vi "Launch Test.vi"(5 "timeout ms (-1)":i32=-1, 6 "Station":T1(ring), 8 "error in (no error)":errorcluster, 10 "SerialNumber":string[](array[string]), 11 "Sequence":string) -> (0 "error out":errorcluster)   [LabVIEW 2019, in "Test Bench Tools.lvlib"]
uses:
  Test Bench Tools.lvlib
  TB Global 1.vi
  <resource>/objmgr/ni.dex.rc
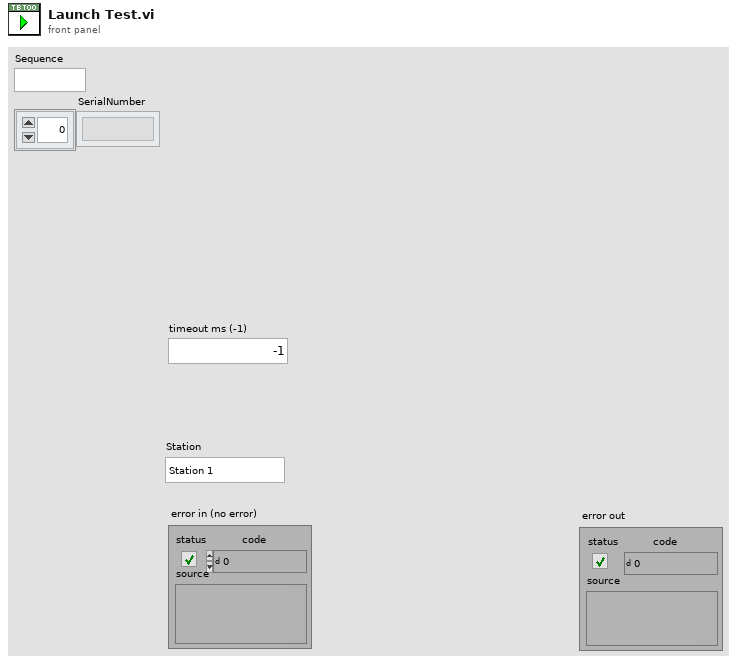
[diagram p1: front panel]
types:
  T1 = enum16{"Station 1", "Station 2", "Station 3", "Station 4"}
  T2 = cluster{"Sequence":string, "SerialNumber":string[]}
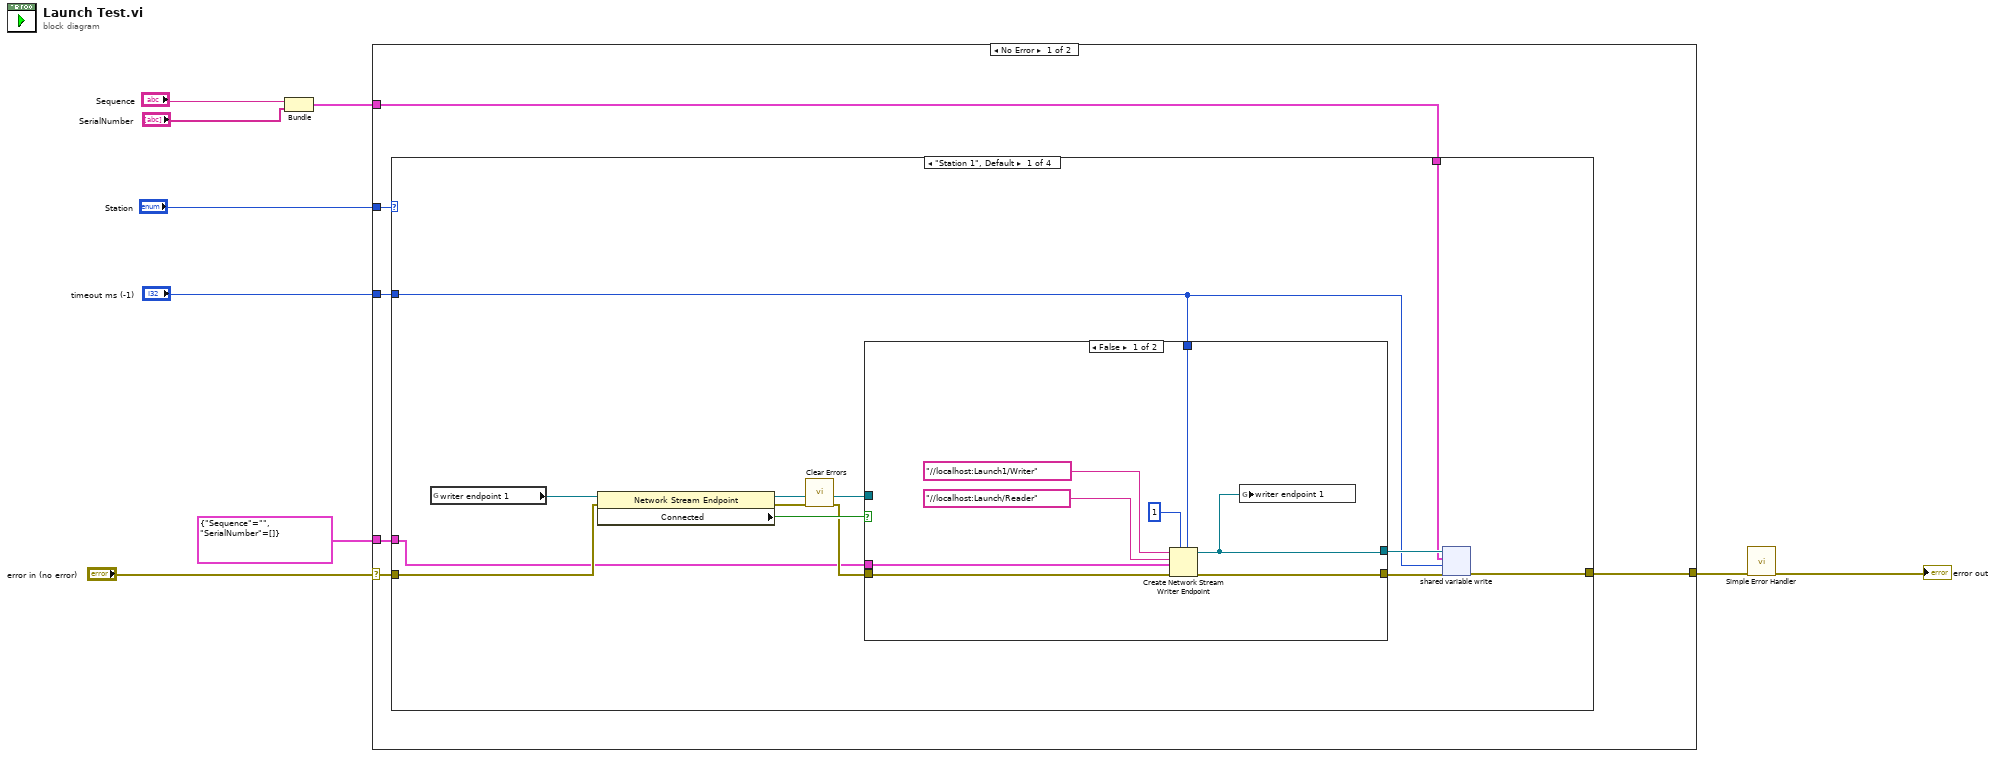
[diagram p0: block diagram]
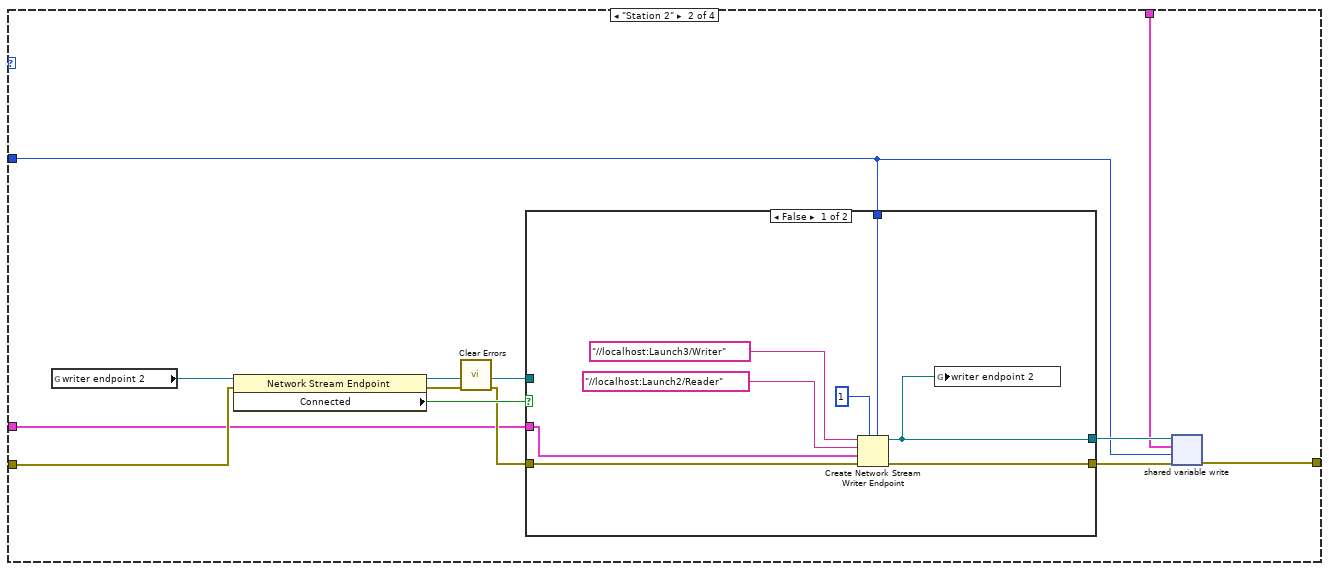
[diagram p3: hidden frame]
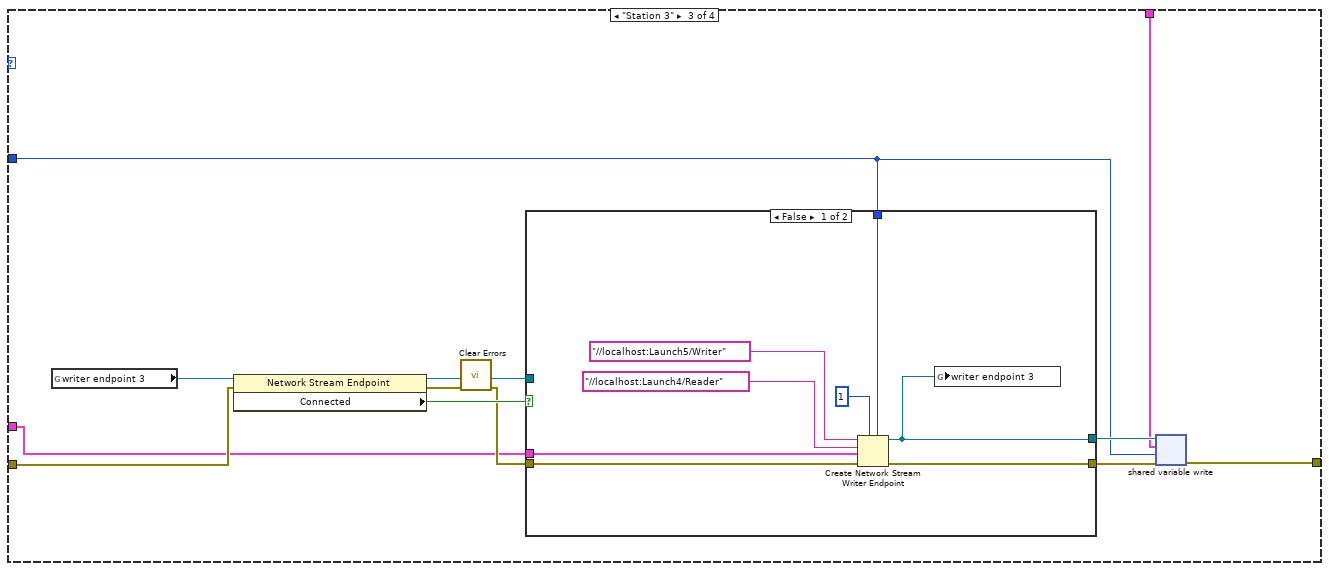
[diagram p5: hidden frame]
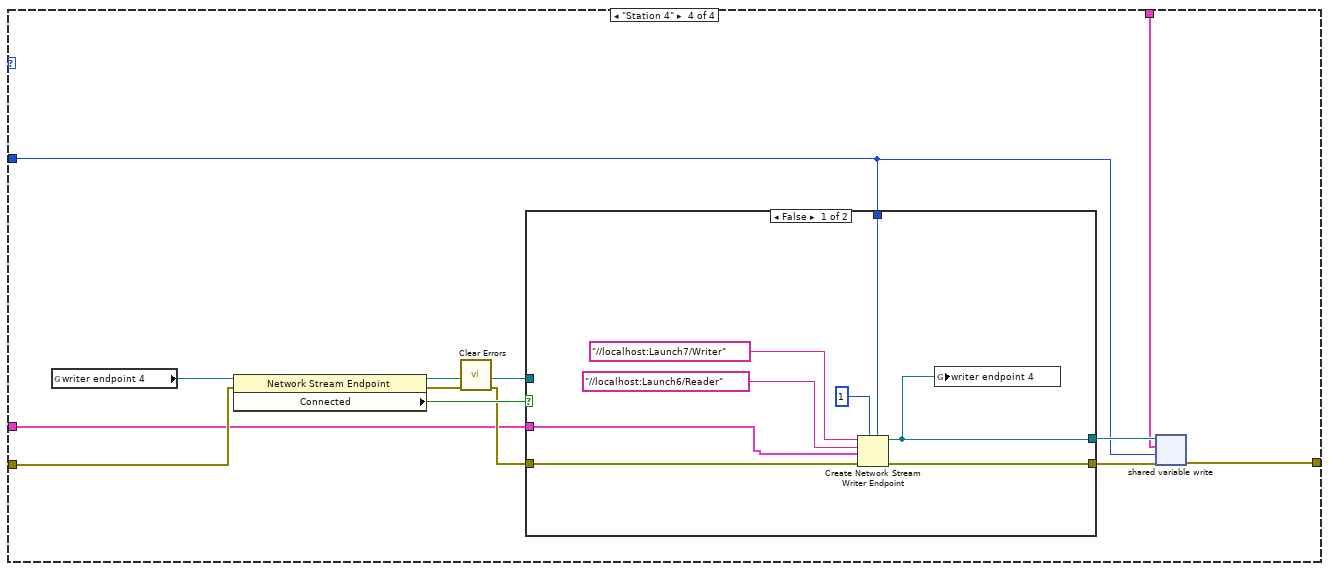
[diagram p7: hidden frame]
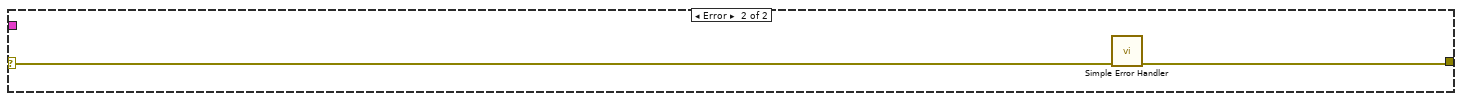
[diagram p9: hidden frame]
diagram:
  n1 = Bundle("Sequence"="Sequence", "SerialNumber"="SerialNumber") -> (w8:T2)  [unwired: 1 in]
  n2 = case shown="No Error" "error in (no error)" {
    selector: "error in (no error)" -> [w14 w105]
    tunnel: "timeout ms (-1)" -> [w13 _]
    tunnel: w8 -> [w12 _]
    tunnel: [w15 w104] -> w7
    tunnel: "Station" -> [w11 _]
    tunnel: T2 {"Sequence"="", "SerialNumber"=[]} -> [w10 _]
    frame No Error {
      n3 = case shown="\"Station 1\", Default" w11 {
        tunnel: [w21 w43 w65 w87] -> w15
        tunnel: w14 -> [w20 w42 w64 w86]
        tunnel: w13 -> [w18 w40 w62 w84]
        tunnel: w12 -> [w17 w39 w61 w83]
        tunnel: w10 -> [w16 w38 w60 w82]
        frame "Station 1", Default {
          n4 = global read "TB Global 1.vi" "writer endpoint 1"() -> (w25:refnum<k21>)
          n5 = property class="Network Stream Endpoint"(reference=w25, error in=w20) -> (reference out=w22:refnum<k21>, error out=w24:errorcluster, "Connected"=w23:bool)
          n6 = call <vilib>:"Clear Errors.vi"("error in (no error)"=w24) -> ("error out"=w19:errorcluster)  [unwired: 5 in, 1 out]
          n7 = case shown="False" w23 {
            tunnel: [w28 w37] -> w27
            tunnel: [w30 w36] -> w26
            tunnel: w19 -> [w32 w36]
            tunnel: w22 -> [_ w37]
            tunnel: w18 -> [w31 _]
            tunnel: w16 -> [w29 _]
            frame False {
              n8 = Create Network Stream Writer Endpoint(5:w31, 7:1 ("writer buffer size"), 8:w32, 9:w29, 10:"//localhost:Launch/Reader" ("reader name"), 11:"//localhost:Launch1/Writer" ("reader name")) -> (0:w30:errorcluster, 3:w28:refnum<k21>)  [unwired: 1 in]
              n9 = global write "TB Global 1.vi" "writer endpoint 1"(w28) -> ()
            }
            frame True {
            }
          }
          n10 = shared-variable-write(w27, w26, w17, w18) -> (w21:errorcluster)  [unwired: 2 out]
        }
        frame "Station 2" {
          n11 = global read "TB Global 1.vi" "writer endpoint 2"() -> (w47:refnum<k21>)
          n12 = property class="Network Stream Endpoint"(reference=w47, error in=w42) -> (reference out=w44:refnum<k21>, error out=w46:errorcluster, "Connected"=w45:bool)
          n13 = call <vilib>:"Clear Errors.vi"("error in (no error)"=w46) -> ("error out"=w41:errorcluster)  [unwired: 5 in, 1 out]
          n14 = case shown="False" w45 {
            tunnel: [w51 w59] -> w49
            tunnel: [w52 w58] -> w48
            tunnel: w41 -> [w54 w58]
            tunnel: w44 -> [_ w59]
            tunnel: w40 -> [w53 _]
            tunnel: w38 -> [w50 _]
            frame False {
              n15 = Create Network Stream Writer Endpoint(5:w53, 7:1 ("writer buffer size"), 8:w54, 9:w50, 10:"//localhost:Launch2/Reader" ("reader name"), 11:"//localhost:Launch3/Writer" ("reader name")) -> (0:w52:errorcluster, 3:w51:refnum<k21>)  [unwired: 1 in]
              n16 = global write "TB Global 1.vi" "writer endpoint 2"(w51) -> ()
            }
            frame True {
            }
          }
          n17 = shared-variable-write(w49, w48, w39, w40) -> (w43:errorcluster)  [unwired: 2 out]
        }
        frame "Station 3" {
          n18 = global read "TB Global 1.vi" "writer endpoint 3"() -> (w69:refnum<k21>)
          n19 = property class="Network Stream Endpoint"(reference=w69, error in=w64) -> (reference out=w66:refnum<k21>, error out=w68:errorcluster, "Connected"=w67:bool)
          n20 = call <vilib>:"Clear Errors.vi"("error in (no error)"=w68) -> ("error out"=w63:errorcluster)  [unwired: 5 in, 1 out]
          n21 = case shown="False" w67 {
            tunnel: [w73 w81] -> w71
            tunnel: [w74 w80] -> w70
            tunnel: w63 -> [w76 w80]
            tunnel: w66 -> [_ w81]
            tunnel: w62 -> [w75 _]
            tunnel: w60 -> [w72 _]
            frame False {
              n22 = Create Network Stream Writer Endpoint(5:w75, 7:1 ("writer buffer size"), 8:w76, 9:w72, 10:"//localhost:Launch4/Reader" ("reader name"), 11:"//localhost:Launch5/Writer" ("reader name")) -> (0:w74:errorcluster, 3:w73:refnum<k21>)  [unwired: 1 in]
              n23 = global write "TB Global 1.vi" "writer endpoint 3"(w73) -> ()
            }
            frame True {
            }
          }
          n24 = shared-variable-write(w71, w70, w61, w62) -> (w65:errorcluster)  [unwired: 2 out]
        }
        frame "Station 4" {
          n25 = global read "TB Global 1.vi" "writer endpoint 4"() -> (w91:refnum<k21>)
          n26 = property class="Network Stream Endpoint"(reference=w91, error in=w86) -> (reference out=w88:refnum<k21>, error out=w90:errorcluster, "Connected"=w89:bool)
          n27 = call <vilib>:"Clear Errors.vi"("error in (no error)"=w90) -> ("error out"=w85:errorcluster)  [unwired: 5 in, 1 out]
          n28 = case shown="False" w89 {
            tunnel: [w95 w103] -> w93
            tunnel: [w96 w102] -> w92
            tunnel: w85 -> [w98 w102]
            tunnel: w88 -> [_ w103]
            tunnel: w84 -> [w97 _]
            tunnel: w82 -> [w94 _]
            frame False {
              n29 = Create Network Stream Writer Endpoint(5:w97, 7:1 ("writer buffer size"), 8:w98, 9:w94, 10:"//localhost:Launch6/Reader" ("reader name"), 11:"//localhost:Launch7/Writer" ("reader name")) -> (0:w96:errorcluster, 3:w95:refnum<k21>)  [unwired: 1 in]
              n30 = global write "TB Global 1.vi" "writer endpoint 4"(w95) -> ()
            }
            frame True {
            }
          }
          n31 = shared-variable-write(w93, w92, w83, w84) -> (w87:errorcluster)  [unwired: 2 out]
        }
      }
    }
    frame Error {
      n32 = call <vilib>:"Simple Error Handler.vi"("error in (no error)"=w105) -> ("error out"=w104:errorcluster)  [unwired: 4 in, 4 out]
    }
  }
  n33 = call <vilib>:"Simple Error Handler.vi"("error in (no error)"=w7) -> ("error out"=→"error out":errorcluster)  [unwired: 4 in, 4 out]
